vi "Send Telnet Message.vi"(8 "error in":errorcluster, 10 "Message In":string, 11 "Telnet V2 in":refnum<class "Telnet V2.lvclass">) -> (0 "error out":errorcluster)   [LabVIEW 2018, in "Telnet V2.lvlib" / "Telnet V2.lvclass"]
uses:
  Telnet V2.lvclass
  Telnet V2.lvclass/Telnet V2.ctl
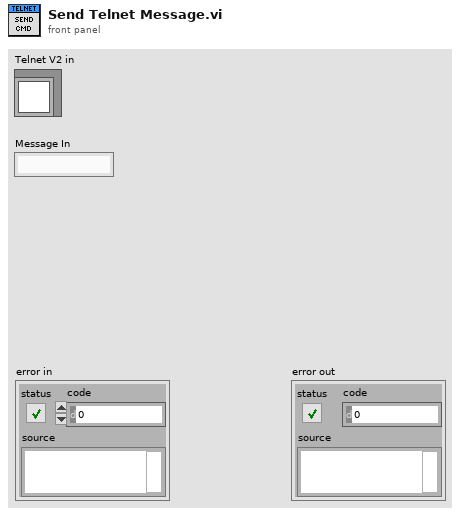
[diagram p1: front panel]
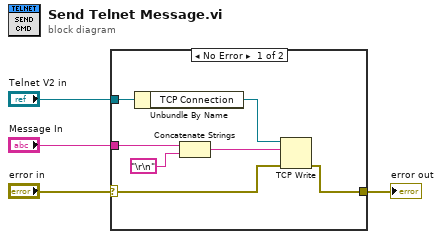
[diagram p0: block diagram]
diagram:
  n1 = case shown="No Error" "error in" {
    selector: "error in" -> [w7 w12]
    tunnel: "Telnet V2 in" -> [w9 _]
    tunnel: "Message In" -> [w10 _]
    tunnel: [w6 w12] -> w1
    frame No Error {
      n2 = Unbundle By Name(w9) -> ("TCP Connection"=w8:refnum<k5>)
      n3 = Concatenate Strings(w10, "\r\n") -> (w5:string)
      n4 = TCP Write(connection ID=w8, data in=w5, error in (no error)=w7) -> (error out=w6:errorcluster)  [unwired: 1 in, 2 out]
    }
    frame Error {
    }
  }
  "error out" <- w1
